vi "AIT 1553 - Load Database - Dynamic.vi"(8 "error in (no error)":errorcluster, 10 "Simulyzer File Path":path, 11 "Node Ptr":u64 format="%.0x") -> (0 "error out":errorcluster)   [LabVIEW 2013]
uses:
  <vilib>/NI Veristand/Custom Device API/Custom Device Item Ref.ctl
  <vilib>/NI Veristand/Custom Device API/Set Item Property (Path).vi
  <vilib>/NI Veristand/Custom Device API/Set Item Property (String).vi
  <vilib>/NI Veristand/Custom Device API/Get Item Property (Path).vi
  Controls and Global/Global.vi
  <vilib>/NI Veristand/Custom Device API/Custom Device API.lvlib
  AIT 664 Custom Device.lvlib
panel:
  out "Item Ref out 2":T1=18446744073709551615 format="%.0x"
  out "selected path 2":path
  out "Item Ref out":T1=18446744073709551615 format="%.0x"
  out "Node Ptr dup":u64
  out "empty path":bool
  out "Win File Path":string
  in  "Tag":string
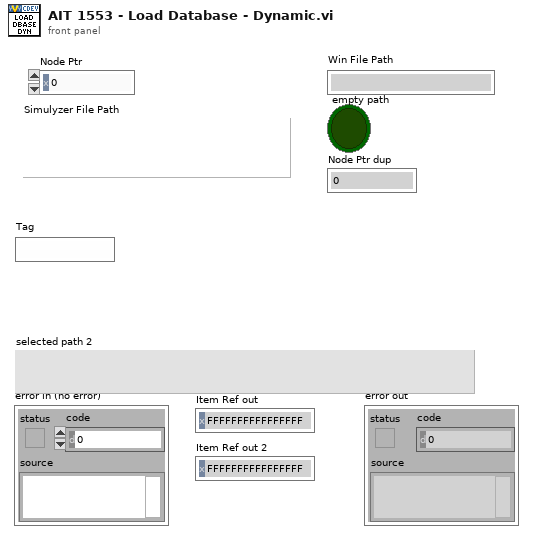
[diagram p1: front panel]
types:
  T1 = typedef "Custom Device API.lvlib/Custom Device Item Ref.ctl" = u64
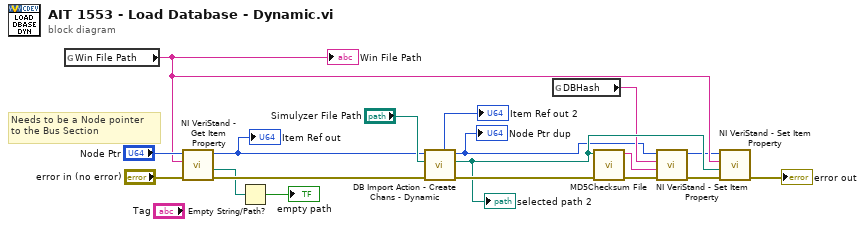
[diagram p0: block diagram]
diagram:
  # "Needs to be a Node pointer \nto the Bus Section"
  n1 = global read "Global.vi" "Win File Path"() -> (w10:string)
  "Win File Path" <- w10
  n2 = call-poly <vilib>:"NI VeriStand - Get Item Property.vi"("error in (no error)"="error in (no error)", "Property Name"=w10, "Item Ref in"="Node Ptr") -> ("error out"=w11:errorcluster, "Value"=w8:path, "Item Ref out"=w12:T1)  [unwired: 5 in, 1 out]
  "Item Ref out" <- w12
  n3 = Empty String/Path?(string/path=w8) -> (empty?=→"empty path":bool)
  n4 = call "DB Import Action - Create Chans - Dynamic.vi"("error in (no error)"=w11, "selected path"="Simulyzer File Path", "Node Ptr"=w12) -> ("error out"=w15:errorcluster, "selected path out"=w14:path, "Node Ptr dup"=w1:u64, "Item Ref"=→"Item Ref out 2":T1)  [unwired: 5 in]
  "Node Ptr dup" <- w1
  "selected path 2" <- w14
  n5 = global read "Global.vi" "DBHash"() -> (w13:string)
  n6 = call <vilib>:"MD5Checksum File.vi"("error in (no error)"=w15, "Path"=w14) -> ("error out"=w4:errorcluster, "MD5 message-digest"=w3:string)  [unwired: 8 in]
  n7 = call-poly <vilib>:"NI VeriStand - Set Item Property.vi"("error in (no error)"=w4, "Value"=w3, "Property Name"=w13, "Item Ref in"=w1) -> ("error out"=w5:errorcluster, "Item Ref out"=w6:T1)  [unwired: 5 in, 1 out]
  n8 = call-poly <vilib>:"NI VeriStand - Set Item Property.vi"("error in (no error)"=w5, "Value"=w14, "Property Name"=w10, "Item Ref in"=w6) -> ("error out"=→"error out":errorcluster)  [unwired: 5 in, 2 out]
